vi "Memory Functional Global.vi"(7 "Memory Option":T1, 8 "error in (no error)":errorcluster, 10 "Number In":ext, 11 "'M' Refnum":refnum<vi>) -> (0 "error out":errorcluster, 2 "Number Out":ext)   [LabVIEW 2013]
doc: "This Functional Global Variable provides storage, access, and modifications to the number stored in the Calculator's memory.\n\nAuthor: Erik Johnson, National Instruments"
uses:
  Custom Controls/Memory Options.ctl
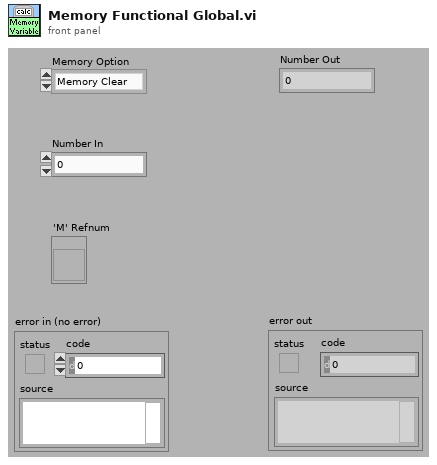
[diagram p1: front panel]
types:
  T1 = typedef "Memory Options.ctl" = enum16{"Memory Clear", "Memory Recall", "Memory Store", "Memory Add"}
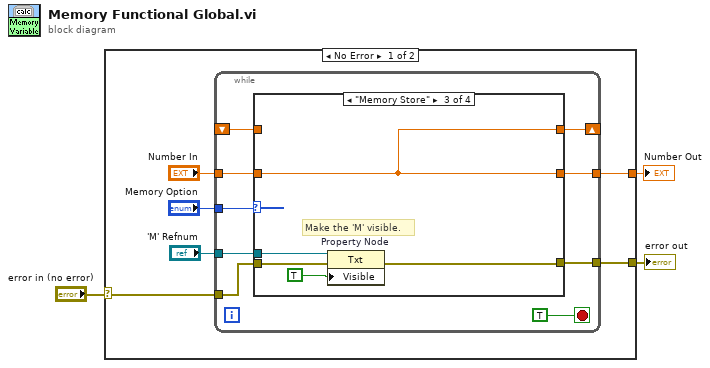
[diagram p0: block diagram]
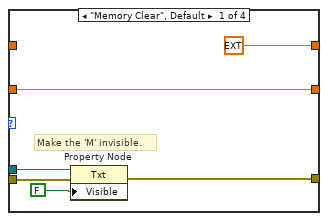
[diagram p2: hidden frame]
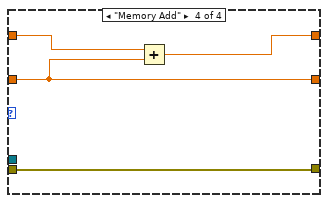
[diagram p4: hidden frame]
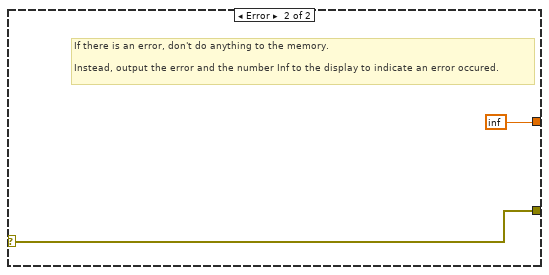
[diagram p5: hidden frame]
diagram:
  n1 = case shown="No Error" "error in (no error)" {
    selector: "error in (no error)" -> [w4 w37]
    tunnel: [w7 inf] -> w3
    tunnel: [w5 w37] -> w2
    frame No Error {
      n2 = while {
        tunnel: "Memory Option" -> [w17]
        shift-right: [w15] -> _
        shift-left: _ -> [w14]
        tunnel: "Number In" -> [w16]
        tunnel: [w13] -> w7
        tunnel: "'M' Refnum" -> [w12]
        tunnel: w4 -> [w11]
        tunnel: [w10] -> w5
        stop <- TRUE stop-if-true
        n3 = case shown="\"Memory Store\"" w17 {
          tunnel: w16 -> [w23 _ w31 w33]
          tunnel: [ext 0.0 w26 w31 w34] -> w15
          tunnel: w14 -> [_ w26 _ w35]
          tunnel: [w23 w26 w31 w33] -> w13
          tunnel: w12 -> [w21 _ w29 _]
          tunnel: w11 -> [w20 w25 w28 w32]
          tunnel: [w19 w25 w27 w32] -> w10
          frame "Memory Clear", Default {
            # "Make the 'M' invisible."
            n4 = property on="Property Node" class="Txt"(reference=w21, error in=w20, "Visible"=FALSE) -> (error out=w19:errorcluster)  [unwired: 1 out]
          }
          frame "Memory Recall" {
          }
          frame "Memory Store" {
            # "Make the 'M' visible."
            n5 = property on="Property Node" class="Txt"(reference=w29, error in=w28, "Visible"=TRUE) -> (error out=w27:errorcluster)  [unwired: 1 out]
          }
          frame "Memory Add" {
            n6 = Add(x=w35, y=w33) -> (x+y=w34:ext)
          }
        }
      }
    }
    frame Error {
      # "If there is an error, don't do anything to the memory.\n\nInstead, output the error and the number Inf to the display to indicate an error occured."
    }
  }
  "Number Out" <- w3
  "error out" <- w2
